vi "List Software.vi"() -> ()   [LabVIEW 2016]
uses:
  <vilib>/nisyscfg/Software 1.2.ctl
  <vilib>/nisyscfg/Component Type.ctl
  <vilib>/nisyscfg/Component Types.ctl
  <vilib>/nisyscfg/Get Installed Components.vi
  <vilib>/nisyscfg/nisyscfg.lvlib
panel:
  in  "Item Types (all visible)":T1 items=["all visible", "all including hidden", "standard only", "startup only"]
  out "Error Out":errorcluster
  out "Software Components":T2[](array[typedef]) {"component type" items=["standard", "hidden", "system", "unknown", "startup", "image"]}
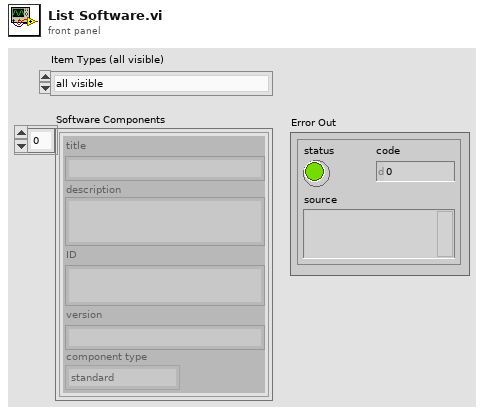
[diagram p1: front panel]
types:
  T1 = typedef "nisyscfg.lvlib/Component Types.ctl" = u32
  T2 = typedef "nisyscfg.lvlib/Software 1.2.ctl" = cluster{"title":string, "description":string, "ID":string, "version":string, "component type":T3}
  T3 = typedef "nisyscfg.lvlib/Component Type.ctl" = u32
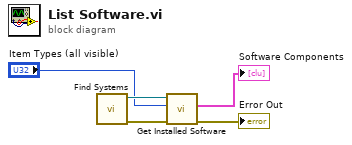
[diagram p0: block diagram]
diagram:
  n1 = call <vilib>:"Find Systems.vi"() -> ("error out"=w3:errorcluster, "Session out"=w5:refnum<k21>)  [unwired: 9 in, 1 out]
  n2 = call-poly <vilib>:"Get Installed Software.vi"("error in (no error)"=w3, "Item Types (all visible)"="Item Types (all visible)", "Session in"=w5) -> ("error out"=→"Error Out":errorcluster, "Software Components"=→"Software Components":T2[])  [unwired: 6 in, 1 out]
